vi "Mouse Click Event.vi"(8 "错误输入（无错误）":errorcluster, 11 "Mouse Click":T1) -> (0 "错误输出":errorcluster)   [LabVIEW 2012, in "API.lvlib"]
uses:
  API.lvlib
  Mouse_Click.ctl
  Mouse_Event.ctl
  user32.dll
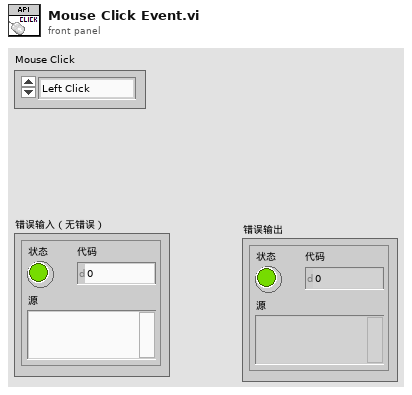
[diagram p1: front panel]
types:
  T1 = typedef "API.lvlib/Mouse_Click.ctl" = enum16{"Left Click", "Left dbClick", "Right Click", "Right dbClick", "Middle Click", "Middle dbClick"}
  T2 = typedef "API.lvlib/Mouse_Event.ctl" = u32
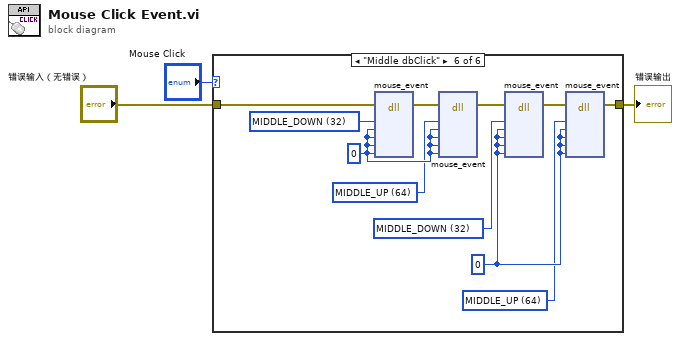
[diagram p0: block diagram]
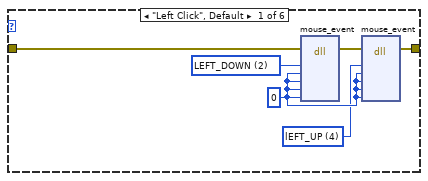
[diagram p2: hidden frame]
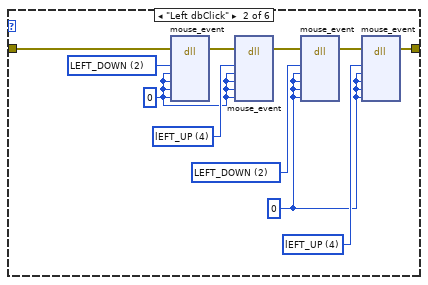
[diagram p3: hidden frame]
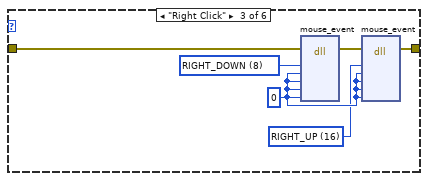
[diagram p4: hidden frame]
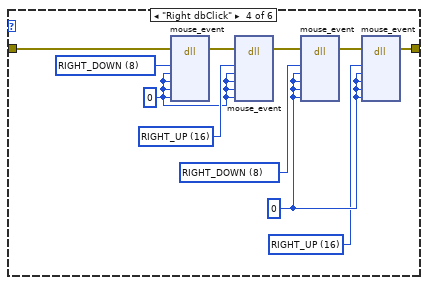
[diagram p5: hidden frame]
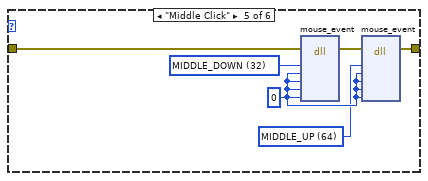
[diagram p6: hidden frame]
diagram:
  n1 = case shown="\"Middle dbClick\"" "Mouse Click" {
    tunnel: "错误输入（无错误）" -> [w9 w16 w22 w27 w39 w50]
    tunnel: [w4 w10 w21 w28 w38 w44] -> w1
    frame "Left Click", Default {
      w5 = T2 4 items=["MOVE"=1, "LEFT_DOWN"=2, "lEFT_UP"=4, "RIGHT_DOWN"=8, "RIGHT_UP"=16, "MIDDLE_DOWN"=32, "MIDDLE_UP"=64, "MOUSE_WHEEL"=128, "ABSOLUTE"=32768] ("文本下拉列表")
      w6 = u32 0 ("dwExtraInfo")
      w7 = T2 2 items=["MOVE"=1, "LEFT_DOWN"=2, "lEFT_UP"=4, "RIGHT_DOWN"=8, "RIGHT_UP"=16, "MIDDLE_DOWN"=32, "MIDDLE_UP"=64, "MOUSE_WHEEL"=128, "ABSOLUTE"=32768] ("文本下拉列表")
      n2 = dll-call lib="user32.dll" fn="mouse_event"(error in=w9, "dwFlags"=w7, "dx"=w6, "dy"=w6, "dwData"=w6, "dwExtraInfo"=w6) -> (error out=w8:errorcluster)  [unwired: 8 in, 1 out]
      n3 = dll-call lib="user32.dll" fn="mouse_event"(error in=w8, "dwFlags"=w5, "dx"=w6, "dy"=w6, "dwData"=w6, "dwExtraInfo"=w6) -> (error out=w4:errorcluster)  [unwired: 8 in, 1 out]
    }
    frame "Left dbClick" {
      w15 = T2 4 items=["MOVE"=1, "LEFT_DOWN"=2, "lEFT_UP"=4, "RIGHT_DOWN"=8, "RIGHT_UP"=16, "MIDDLE_DOWN"=32, "MIDDLE_UP"=64, "MOUSE_WHEEL"=128, "ABSOLUTE"=32768] ("文本下拉列表")
      w14 = u32 0 ("dwExtraInfo")
      w13 = T2 2 items=["MOVE"=1, "LEFT_DOWN"=2, "lEFT_UP"=4, "RIGHT_DOWN"=8, "RIGHT_UP"=16, "MIDDLE_DOWN"=32, "MIDDLE_UP"=64, "MOUSE_WHEEL"=128, "ABSOLUTE"=32768] ("文本下拉列表")
      w20 = T2 4 items=["MOVE"=1, "LEFT_DOWN"=2, "lEFT_UP"=4, "RIGHT_DOWN"=8, "RIGHT_UP"=16, "MIDDLE_DOWN"=32, "MIDDLE_UP"=64, "MOUSE_WHEEL"=128, "ABSOLUTE"=32768] ("文本下拉列表")
      w19 = u32 0 ("dwExtraInfo")
      w18 = T2 2 items=["MOVE"=1, "LEFT_DOWN"=2, "lEFT_UP"=4, "RIGHT_DOWN"=8, "RIGHT_UP"=16, "MIDDLE_DOWN"=32, "MIDDLE_UP"=64, "MOUSE_WHEEL"=128, "ABSOLUTE"=32768] ("文本下拉列表")
      n4 = dll-call lib="user32.dll" fn="mouse_event"(error in=w16, "dwFlags"=w18, "dx"=w19, "dy"=w19, "dwData"=w19, "dwExtraInfo"=w19) -> (error out=w17:errorcluster)  [unwired: 8 in, 1 out]
      n5 = dll-call lib="user32.dll" fn="mouse_event"(error in=w17, "dwFlags"=w20, "dx"=w19, "dy"=w19, "dwData"=w19, "dwExtraInfo"=w19) -> (error out=w11:errorcluster)  [unwired: 8 in, 1 out]
      n6 = dll-call lib="user32.dll" fn="mouse_event"(error in=w11, "dwFlags"=w13, "dx"=w14, "dy"=w14, "dwData"=w14, "dwExtraInfo"=w14) -> (error out=w12:errorcluster)  [unwired: 8 in, 1 out]
      n7 = dll-call lib="user32.dll" fn="mouse_event"(error in=w12, "dwFlags"=w15, "dx"=w14, "dy"=w14, "dwData"=w14, "dwExtraInfo"=w14) -> (error out=w10:errorcluster)  [unwired: 8 in, 1 out]
    }
    frame "Right Click" {
      w23 = T2 16 items=["MOVE"=1, "LEFT_DOWN"=2, "lEFT_UP"=4, "RIGHT_DOWN"=8, "RIGHT_UP"=16, "MIDDLE_DOWN"=32, "MIDDLE_UP"=64, "MOUSE_WHEEL"=128, "ABSOLUTE"=32768] ("文本下拉列表")
      w24 = u32 0 ("dwExtraInfo")
      w25 = T2 8 items=["MOVE"=1, "LEFT_DOWN"=2, "lEFT_UP"=4, "RIGHT_DOWN"=8, "RIGHT_UP"=16, "MIDDLE_DOWN"=32, "MIDDLE_UP"=64, "MOUSE_WHEEL"=128, "ABSOLUTE"=32768] ("文本下拉列表")
      n8 = dll-call lib="user32.dll" fn="mouse_event"(error in=w22, "dwFlags"=w25, "dx"=w24, "dy"=w24, "dwData"=w24, "dwExtraInfo"=w24) -> (error out=w26:errorcluster)  [unwired: 8 in, 1 out]
      n9 = dll-call lib="user32.dll" fn="mouse_event"(error in=w26, "dwFlags"=w23, "dx"=w24, "dy"=w24, "dwData"=w24, "dwExtraInfo"=w24) -> (error out=w21:errorcluster)  [unwired: 8 in, 1 out]
    }
    frame "Right dbClick" {
      w30 = T2 16 items=["MOVE"=1, "LEFT_DOWN"=2, "lEFT_UP"=4, "RIGHT_DOWN"=8, "RIGHT_UP"=16, "MIDDLE_DOWN"=32, "MIDDLE_UP"=64, "MOUSE_WHEEL"=128, "ABSOLUTE"=32768] ("文本下拉列表")
      w31 = u32 0 ("dwExtraInfo")
      w32 = T2 8 items=["MOVE"=1, "LEFT_DOWN"=2, "lEFT_UP"=4, "RIGHT_DOWN"=8, "RIGHT_UP"=16, "MIDDLE_DOWN"=32, "MIDDLE_UP"=64, "MOUSE_WHEEL"=128, "ABSOLUTE"=32768] ("文本下拉列表")
      w37 = T2 16 items=["MOVE"=1, "LEFT_DOWN"=2, "lEFT_UP"=4, "RIGHT_DOWN"=8, "RIGHT_UP"=16, "MIDDLE_DOWN"=32, "MIDDLE_UP"=64, "MOUSE_WHEEL"=128, "ABSOLUTE"=32768] ("文本下拉列表")
      w36 = u32 0 ("dwExtraInfo")
      w35 = T2 8 items=["MOVE"=1, "LEFT_DOWN"=2, "lEFT_UP"=4, "RIGHT_DOWN"=8, "RIGHT_UP"=16, "MIDDLE_DOWN"=32, "MIDDLE_UP"=64, "MOUSE_WHEEL"=128, "ABSOLUTE"=32768] ("文本下拉列表")
      n10 = dll-call lib="user32.dll" fn="mouse_event"(error in=w27, "dwFlags"=w35, "dx"=w36, "dy"=w36, "dwData"=w36, "dwExtraInfo"=w36) -> (error out=w34:errorcluster)  [unwired: 8 in, 1 out]
      n11 = dll-call lib="user32.dll" fn="mouse_event"(error in=w34, "dwFlags"=w37, "dx"=w36, "dy"=w36, "dwData"=w36, "dwExtraInfo"=w36) -> (error out=w29:errorcluster)  [unwired: 8 in, 1 out]
      n12 = dll-call lib="user32.dll" fn="mouse_event"(error in=w29, "dwFlags"=w32, "dx"=w31, "dy"=w31, "dwData"=w31, "dwExtraInfo"=w31) -> (error out=w33:errorcluster)  [unwired: 8 in, 1 out]
      n13 = dll-call lib="user32.dll" fn="mouse_event"(error in=w33, "dwFlags"=w30, "dx"=w31, "dy"=w31, "dwData"=w31, "dwExtraInfo"=w31) -> (error out=w28:errorcluster)  [unwired: 8 in, 1 out]
    }
    frame "Middle Click" {
      w40 = T2 64 items=["MOVE"=1, "LEFT_DOWN"=2, "lEFT_UP"=4, "RIGHT_DOWN"=8, "RIGHT_UP"=16, "MIDDLE_DOWN"=32, "MIDDLE_UP"=64, "MOUSE_WHEEL"=128, "ABSOLUTE"=32768] ("文本下拉列表")
      w41 = u32 0 ("dwExtraInfo")
      w42 = T2 32 items=["MOVE"=1, "LEFT_DOWN"=2, "lEFT_UP"=4, "RIGHT_DOWN"=8, "RIGHT_UP"=16, "MIDDLE_DOWN"=32, "MIDDLE_UP"=64, "MOUSE_WHEEL"=128, "ABSOLUTE"=32768] ("文本下拉列表")
      n14 = dll-call lib="user32.dll" fn="mouse_event"(error in=w39, "dwFlags"=w42, "dx"=w41, "dy"=w41, "dwData"=w41, "dwExtraInfo"=w41) -> (error out=w43:errorcluster)  [unwired: 8 in, 1 out]
      n15 = dll-call lib="user32.dll" fn="mouse_event"(error in=w43, "dwFlags"=w40, "dx"=w41, "dy"=w41, "dwData"=w41, "dwExtraInfo"=w41) -> (error out=w38:errorcluster)  [unwired: 8 in, 1 out]
    }
    frame "Middle dbClick" {
      w46 = T2 64 items=["MOVE"=1, "LEFT_DOWN"=2, "lEFT_UP"=4, "RIGHT_DOWN"=8, "RIGHT_UP"=16, "MIDDLE_DOWN"=32, "MIDDLE_UP"=64, "MOUSE_WHEEL"=128, "ABSOLUTE"=32768] ("文本下拉列表")
      w47 = u32 0 ("dwExtraInfo")
      w48 = T2 32 items=["MOVE"=1, "LEFT_DOWN"=2, "lEFT_UP"=4, "RIGHT_DOWN"=8, "RIGHT_UP"=16, "MIDDLE_DOWN"=32, "MIDDLE_UP"=64, "MOUSE_WHEEL"=128, "ABSOLUTE"=32768] ("文本下拉列表")
      w51 = T2 64 items=["MOVE"=1, "LEFT_DOWN"=2, "lEFT_UP"=4, "RIGHT_DOWN"=8, "RIGHT_UP"=16, "MIDDLE_DOWN"=32, "MIDDLE_UP"=64, "MOUSE_WHEEL"=128, "ABSOLUTE"=32768] ("文本下拉列表")
      w52 = u32 0 ("dwExtraInfo")
      w53 = T2 32 items=["MOVE"=1, "LEFT_DOWN"=2, "lEFT_UP"=4, "RIGHT_DOWN"=8, "RIGHT_UP"=16, "MIDDLE_DOWN"=32, "MIDDLE_UP"=64, "MOUSE_WHEEL"=128, "ABSOLUTE"=32768] ("文本下拉列表")
      n16 = dll-call lib="user32.dll" fn="mouse_event"(error in=w50, "dwFlags"=w53, "dx"=w52, "dy"=w52, "dwData"=w52, "dwExtraInfo"=w52) -> (error out=w54:errorcluster)  [unwired: 8 in, 1 out]
      n17 = dll-call lib="user32.dll" fn="mouse_event"(error in=w54, "dwFlags"=w51, "dx"=w52, "dy"=w52, "dwData"=w52, "dwExtraInfo"=w52) -> (error out=w45:errorcluster)  [unwired: 8 in, 1 out]
      n18 = dll-call lib="user32.dll" fn="mouse_event"(error in=w45, "dwFlags"=w48, "dx"=w47, "dy"=w47, "dwData"=w47, "dwExtraInfo"=w47) -> (error out=w49:errorcluster)  [unwired: 8 in, 1 out]
      n19 = dll-call lib="user32.dll" fn="mouse_event"(error in=w49, "dwFlags"=w46, "dx"=w47, "dy"=w47, "dwData"=w47, "dwExtraInfo"=w47) -> (error out=w44:errorcluster)  [unwired: 8 in, 1 out]
    }
  }
  "错误输出" <- w1
